vi "Main_Interface.vi"   [LabVIEW 2021]
uses:
  <vilib>/Utility/miscctls.llb/LVPointTypeDef.ctl
  Exit Variable.vi
  Settings page.vi
  SETTING CLOSE GLOBEL VARIABLE.vi
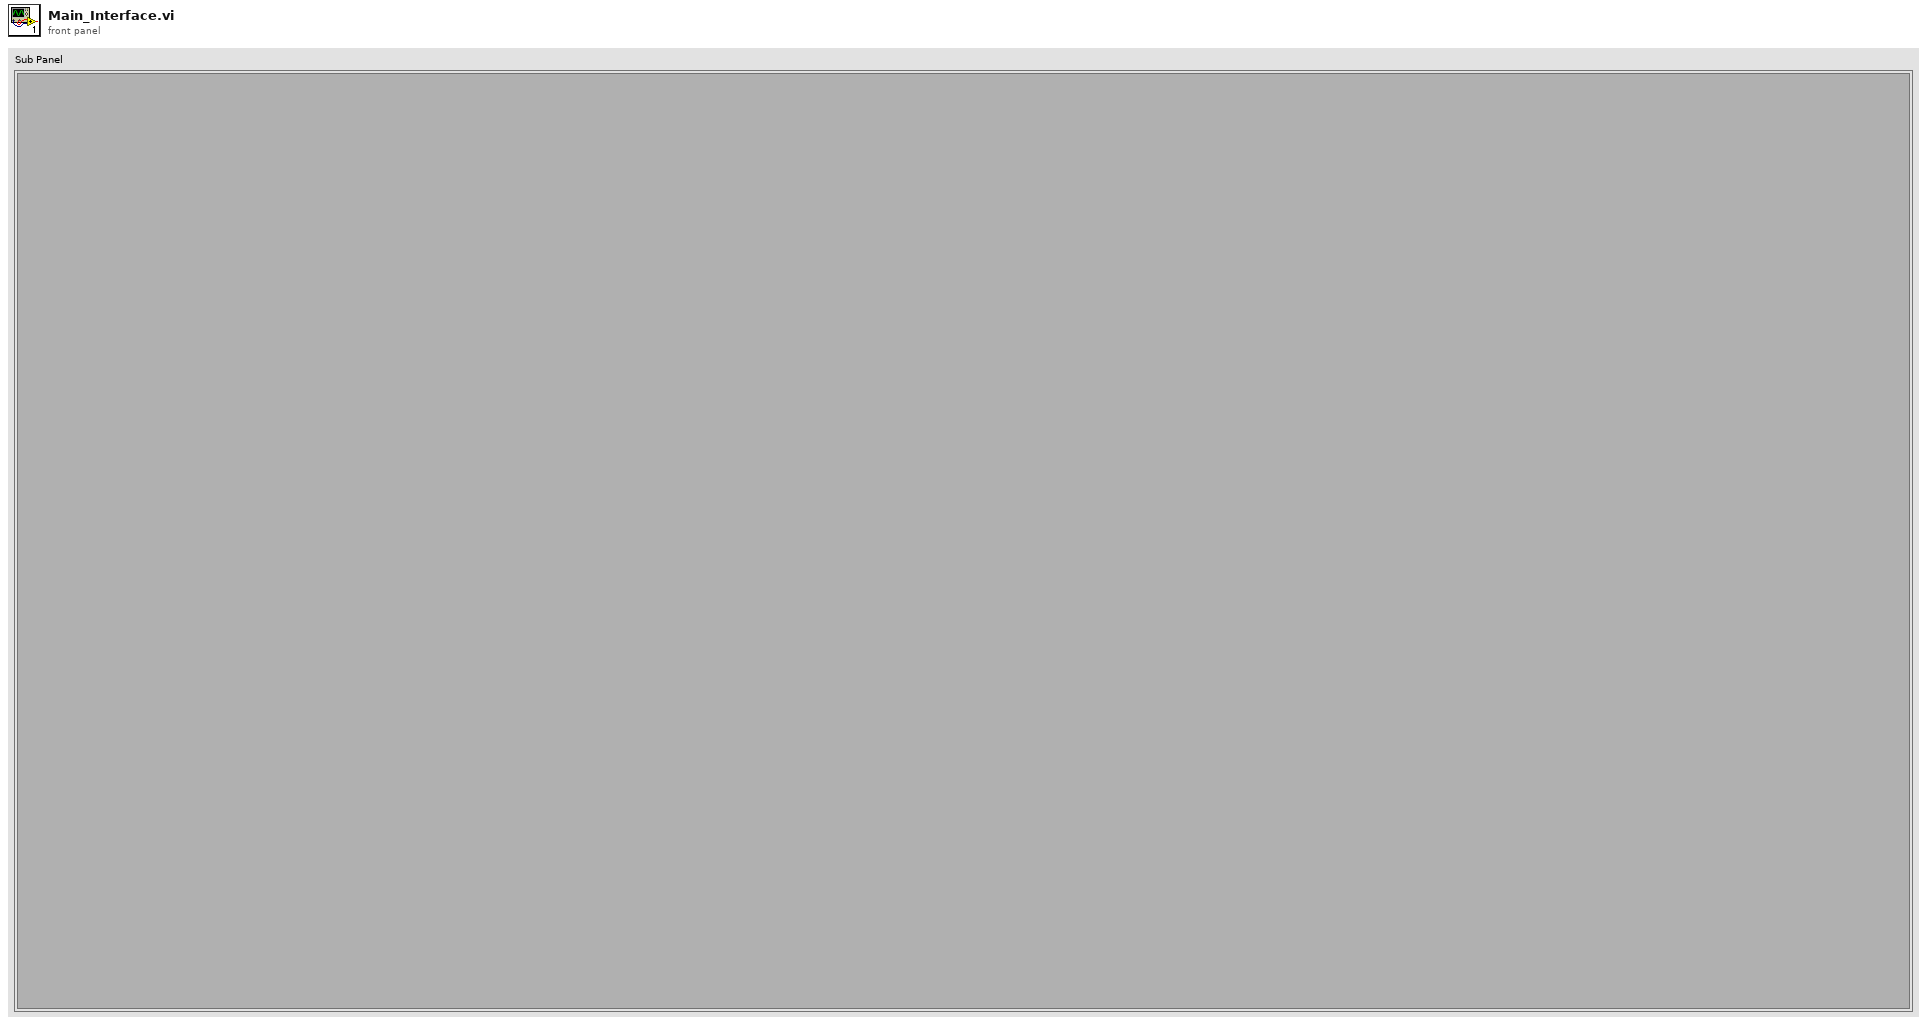
[diagram p1: front panel]
types:
  T1 = typedef "LVPointTypeDef.ctl" = cluster{"Horizontal":i16, "Vertical":i16}
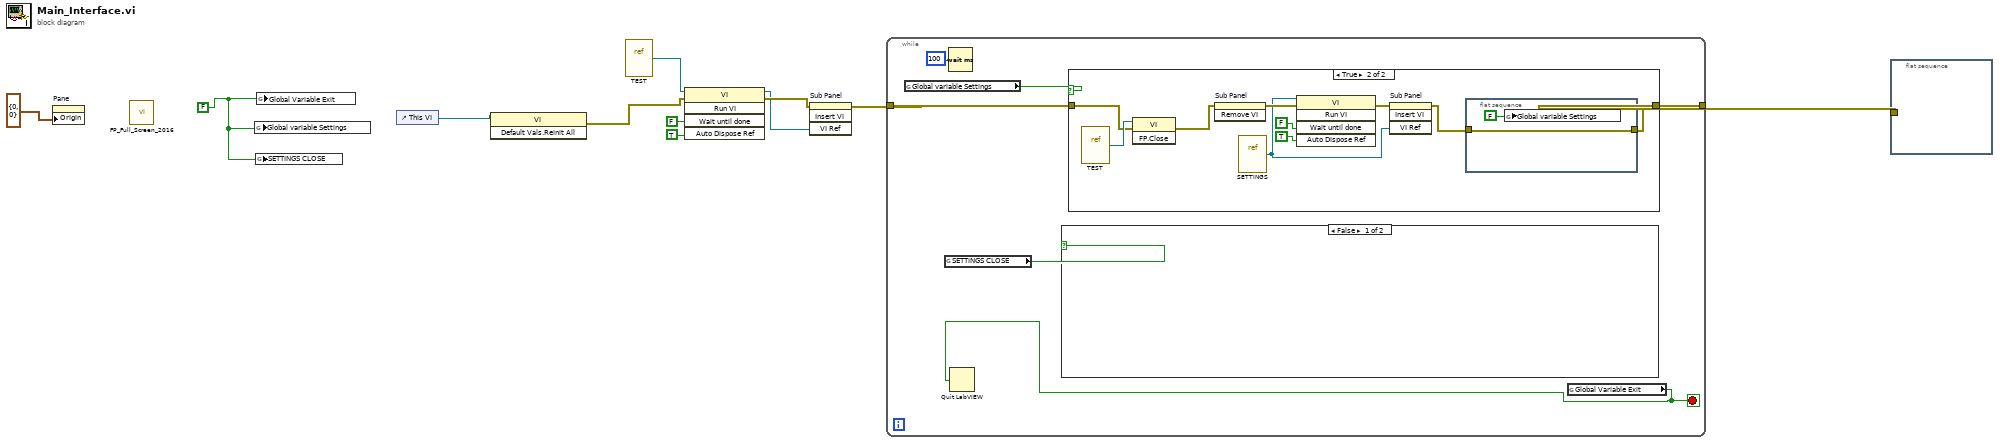
[diagram p0: block diagram]
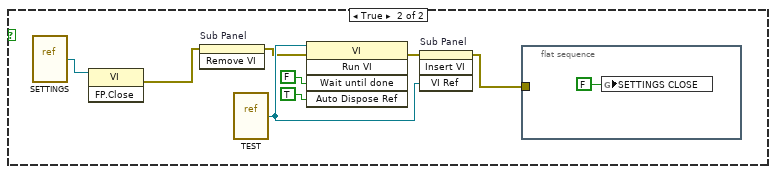
[diagram p2: hidden frame]
diagram:
  w1 = FALSE
  n1 = property on="Pane" class="Pane"("Origin"=T1 {"Horizontal"=0, "Vertical"=0}) -> ()  [unwired: 2 in, 2 out]
  n2 = call "FP_Full_Screen_2016.vi"() -> ()  [unwired: 12 in]
  n3 = global write "Settings page.vi" "Global variable Settings"(w1) -> ()
  n4 = global write "SETTING CLOSE GLOBEL VARIABLE.vi" "SETTINGS CLOSE"(w1) -> ()
  n5 = global write "Exit Variable.vi" "Global Variable Exit"(w1) -> ()
  n6 = control-ref of="This VI"() -> (w7:refnum<vi>)
  n7 = invoke class="VI" method="Default Vals.Reinit All"(reference=w7) -> (error out=w6:errorcluster)  [unwired: 2 in, 2 out]
  n8 = vi-ref "TEST.vi"() -> (w2:refnum<vi>)
  n9 = invoke class="VI" method="Run VI"(reference=w2, error in=w6, "Wait until done"=FALSE ("Wait Until Done"), "Auto Dispose Ref"=TRUE ("Auto Dispose Reference")) -> (reference out=w4:refnum<vi>, error out=w5:errorcluster)  [unwired: 1 in, 3 out]
  n10 = invoke on="Sub Panel" class="SubPnl" method="Insert VI"(error in=w5, "VI Ref"=w4) -> (error out=w8:errorcluster)  [unwired: 2 in, 3 out]
  n11 = while {
    tunnel: w8 -> [w16]
    tunnel: [w15] -> w3
    stop <- w12 stop-if-true
    n12 = global read "Settings page.vi" "Global variable Settings"() -> (w14:bool)
    n13 = global read "SETTING CLOSE GLOBEL VARIABLE.vi" "SETTINGS CLOSE"() -> (w13:bool)
    n14 = Wait (ms)(milliseconds to wait=u32 100) -> ()  [unwired: 1 out]
    n15 = case shown="False" w13 {
      frame False {
      }
      frame True {
        n16 = vi-ref "SETTINGS.vi"() -> (w19:refnum<vi>)
        n17 = invoke class="VI" method="FP.Close"(reference=w19) -> (error out=w18:errorcluster)  [unwired: 2 in, 2 out]
        n18 = invoke on="Sub Panel" class="SubPnl" method="Remove VI"(error in=w18) -> (error out=w20:errorcluster)  [unwired: 2 in, 2 out]
        n19 = vi-ref "TEST.vi"() -> (w22:refnum<vi>)
        n20 = invoke class="VI" method="Run VI"(reference=w22, error in=w20, "Wait until done"=FALSE ("Wait Until Done"), "Auto Dispose Ref"=TRUE ("Auto Dispose Reference")) -> (error out=w23:errorcluster)  [unwired: 1 in, 4 out]
        n21 = invoke on="Sub Panel" class="SubPnl" method="Insert VI"(error in=w23, "VI Ref"=w22) -> (error out=w21:errorcluster)  [unwired: 2 in, 3 out]
        n22 = flat-sequence {
          tunnel: w21 -> [_]
          frame #0 {
            n23 = global write "SETTING CLOSE GLOBEL VARIABLE.vi" "SETTINGS CLOSE"(FALSE ("SETTINGS CLOSE")) -> ()
          }
        }
      }
    }
    n24 = case shown="True" w14 {
      tunnel: w16 -> [w27 w29]
      tunnel: [w27 w31] -> w15
      frame False {
      }
      frame True {
        n25 = vi-ref "TEST.vi"() -> (w30:refnum<vi>)
        n26 = invoke class="VI" method="FP.Close"(reference=w30, error in=w29) -> (error out=w28:errorcluster)  [unwired: 1 in, 2 out]
        n27 = invoke on="Sub Panel" class="SubPnl" method="Remove VI"(error in=w28) -> (error out=w35:errorcluster)  [unwired: 2 in, 2 out]
        n28 = vi-ref "SETTINGS.vi"() -> (w33:refnum<vi>)
        n29 = invoke class="VI" method="Run VI"(reference=w33, error in=w35, "Wait until done"=FALSE ("Wait Until Done"), "Auto Dispose Ref"=TRUE ("Auto Dispose Reference")) -> (error out=w34:errorcluster)  [unwired: 1 in, 4 out]
        n30 = invoke on="Sub Panel" class="SubPnl" method="Insert VI"(error in=w34, "VI Ref"=w33) -> (error out=w32:errorcluster)  [unwired: 2 in, 3 out]
        n31 = flat-sequence {
          tunnel: w32 -> [w38]
          tunnel: [w38] -> w31
          frame #0 {
            n32 = global write "Settings page.vi" "Global variable Settings"(FALSE ("Global variable Settings")) -> ()
          }
        }
      }
    }
    n33 = global read "Exit Variable.vi" "Global Variable Exit"() -> (w12:bool)
    n34 = Quit LabVIEW(quit? (T)=w12) -> ()
  }
  n35 = flat-sequence {
    tunnel: w3 -> [_]
    frame #0 {
    }
  }
